vi "Sequence Engine.vi"(11 "gController in":refnum<class "gController.lvclass">) -> (3 "gController out":refnum<class "gController.lvclass">)   [LabVIEW 2018, in "Controller.lvlib" / "gController.lvclass"]
uses:
  gController.lvclass
  C:/Program Files (x86)/National Instruments/LabVIEW 2018/vi.lib/MSR Consulting, LLC/General Reuse/SuperActor/SuperActor.lvclass
  sequenceState.ctl
  <vilib>/MSR Consulting, LLC/General Reuse/SuperActor/SuperActor.lvclass/SuperActor.ctl
  gController.lvclass/gController.ctl
  <vilib>/MSR Consulting, LLC/General Reuse/SuperActor/Read Log Session.vi
  Read seq_state.vi
  <vilib>/MSR Consulting, LLC/General Reuse/SuperActor/Read CVT Session.vi
  <vilib>/MSR Consulting, LLC/General Reuse/Session APIs/_Session Fwk/Session - Root.lvclass
  <vilib>/MSR Consulting, LLC/General Reuse/Sequence/SEQ/SEQ.lvclass
  <vilib>/MSR Consulting, LLC/General Reuse/Session APIs/Session Log/System Log.lvclass
  Controller.lvlib
  <vilib>/MSR Consulting, LLC/General Reuse/Session APIs/CVT/CVT.lvclass
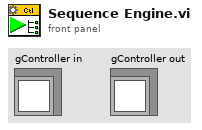
[diagram p1: front panel]
types:
  T1 = typedef "Controller.lvlib/sequenceState.ctl" = enum16{"Run", "Pause", "Reset", "Reload", "Stop"}
  T2 = typedef "Session - Root.lvclass/Session Handle.ctl" = refnum<data-value>
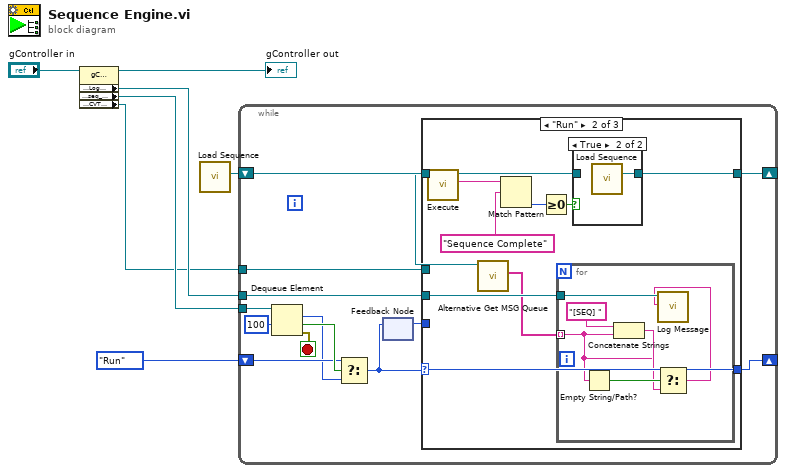
[diagram p0: block diagram]
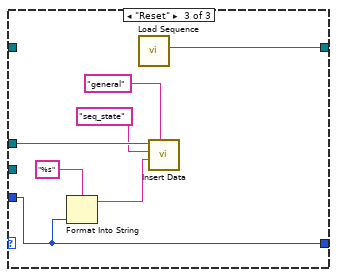
[diagram p4: hidden frame]
diagram:
  n1 = property class="gController"(reference="gController in") -> (reference out=→"gController out":refnum<class "gController.lvclass">, "Accessors:Log Session"=w7:T2, "Accessors:seq_state"=w4:refnum<queue>, "Accessors:CVT Session"=w1:T2)  [unwired: 1 in, 1 out]
  n2 = call "Load Sequence.vi"() -> ("SEQ out"=w3:refnum<class "SEQ.lvclass">)  [unwired: 11 in]
  n3 = while {
    tunnel: w7 -> [w20]
    tunnel: w4 -> [w18]
    shift-right: [w16] -> _
    shift-left: w3 -> [w19]
    shift-right: [w9] -> _
    shift-left: sequenceState."Run" ("sequence state") -> [w14]
    tunnel: w1 -> [w8]
    stop <- w17 stop-if-true
    n4 = Dequeue Element(queue=w18, timeout in ms (-1)=100) -> (element=w13:T1, timed out?=w15:bool, error out=w17:errorcluster)  [unwired: 1 in, 1 out]
    n5 = Select(t=w14, s=w15, f=w13) -> (s? t:f=w11:T1)
    n6 = feedback-in #1(w11) -> ()
    n7 = feedback #1() -> (w10:T1)  [unwired: 1 in]
    n8 = case shown="\"Run\"" w11 {
      selector: w11 -> [w21 w23 _]
      tunnel: w20 -> [_ w32 _]
      tunnel: w19 -> [w22 w31 _]
      tunnel: [w22 w24 w47] -> w16
      tunnel: [w21 w23 w43] -> w9
      tunnel: w10 -> [_ _ w43]
      tunnel: w8 -> [_ _ w46]
      frame "Pause", Default {
      }
      frame "Run" {
        n9 = call-dynamic "Execute.vi"("SEQ in"=w31) -> ("MSG"=w28:string, "SEQ out"=w26:refnum<class "SEQ.lvclass">)  [unwired: 7 in, 2 out]
        n10 = call <vilib>:"Alternative Get MSG Queue.vi"("SEQ in"=w31) -> ("seqMsg"=w29:string[])  [unwired: 9 in, 1 out]
        n11 = Match Pattern(string=w28, regular expression="Sequence Complete" ("y")) -> (offset past match=w27:i32)  [unwired: 1 in, 3 out]
        n12 = Greater Or Equal To 0?(x=w27) -> (x >= 0?=w25:bool)
        n13 = for {
          tunnel: w29 -> [w36] mode=indexing
          tunnel: w32 -> [w40]
          n14 = Empty String/Path?(string/path=w36) -> (empty?=w38:bool)
          n15 = Concatenate Strings("[SEQ] " ("string"), w36) -> (w37:string)
          n16 = Select(t=w36, s=w38, f=w37) -> (s? t:f=w35:string)
          n17 = call <vilib>:"Log Message.vi"("MSG In"=w35, "session in"=w40) -> ()  [unwired: 8 in, 2 out]
        }
        n18 = case shown="True" w25 {
          tunnel: w26 -> [w33 _]
          tunnel: [w33 w34] -> w24
          frame False {
          }
          frame True {
            n19 = call "Load Sequence.vi"() -> ("SEQ out"=w34:refnum<class "SEQ.lvclass">)  [unwired: 11 in]
          }
        }
      }
      frame "Reset" {
        n20 = Format Into String(format string="%s", w43) -> (resulting string=w41:string)  [unwired: 2 in, 1 out]
        n21 = call "Load Sequence.vi"() -> ("SEQ out"=w47:refnum<class "SEQ.lvclass">)  [unwired: 11 in]
        n22 = call <vilib>:"Insert Data.vi"("Group"="general", "Data"=w41, "tag"="seq_state", "CVT Session In"=w46) -> ()  [unwired: 6 in, 2 out]
      }
    }
  }
